vi "Toolkit Binaries Pre-Uninstall Custom Action.vi"(10 "Variant":variant) -> (0 "error out":errorcluster)   [LabVIEW 2020]
uses:
  <vilib>/security/Message Digest/API/Instances/File/SHA-256 File Checksum.vi
  <vilib>/security/Message Digest/API/NI_Message Digest API.lvlib
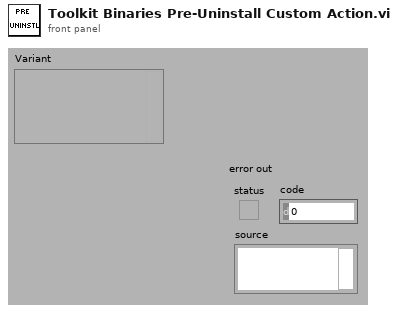
[diagram p1: front panel]
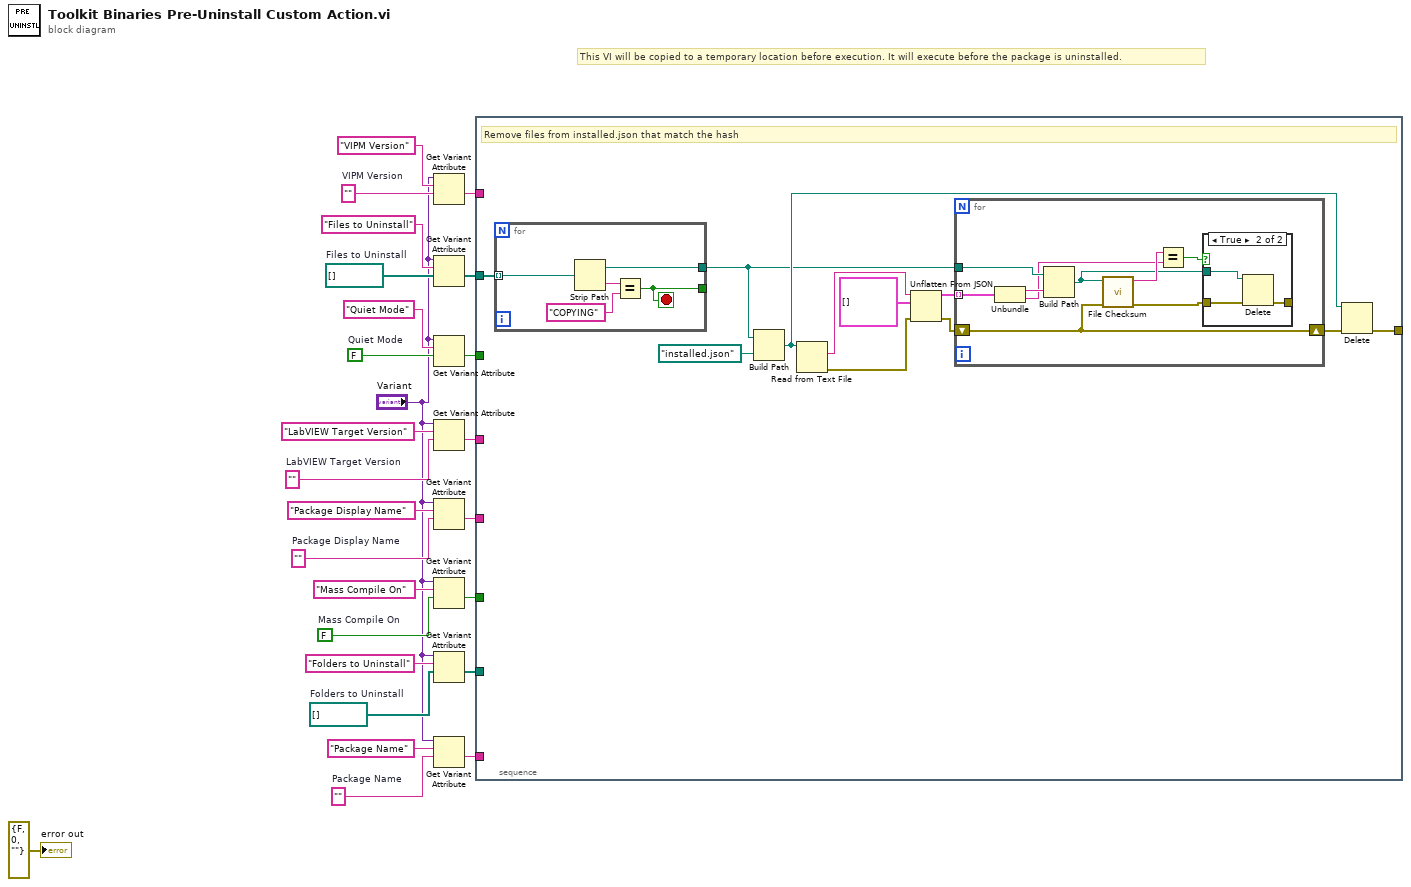
[diagram p0: block diagram]
diagram:
  w3 = path[] []  # Folders to Uninstall
  w7 = path[] []  # Files to Uninstall
  w8 = FALSE  # Mass Compile On
  w9 = ""  # Package Display Name
  w16 = FALSE  # Quiet Mode
  w19 = ""  # VIPM Version
  w21 = ""  # LabVIEW Target Version
  w23 = ""  # Package Name
  # "This VI will be copied to a temporary location before execution. It will execute before the package is uninstalled."
  n1 = Get Variant Attribute(Variant="Variant", name="VIPM Version", default value (empty Variant)=w19) -> (value=w12:string)  [unwired: 1 in, 3 out]
  n2 = Get Variant Attribute(Variant="Variant", name="Files to Uninstall", default value (empty Variant)=w7) -> (value=w5:path[])  [unwired: 1 in, 3 out]
  n3 = Get Variant Attribute(Variant="Variant", name="Quiet Mode", default value (empty Variant)=w16) -> (value=w11:bool)  [unwired: 1 in, 3 out]
  n4 = Get Variant Attribute(Variant="Variant", name="LabVIEW Target Version", default value (empty Variant)=w21) -> (value=w13:string)  [unwired: 1 in, 3 out]
  n5 = Get Variant Attribute(Variant="Variant", name="Package Display Name", default value (empty Variant)=w9) -> (value=w15:string)  [unwired: 1 in, 3 out]
  n6 = Get Variant Attribute(Variant="Variant", name="Mass Compile On", default value (empty Variant)=w8) -> (value=w10:bool)  [unwired: 1 in, 3 out]
  n7 = Get Variant Attribute(Variant="Variant", name="Folders to Uninstall", default value (empty Variant)=w3) -> (value=w2:path[])  [unwired: 1 in, 3 out]
  n8 = Get Variant Attribute(Variant="Variant", name="Package Name", default value (empty Variant)=w23) -> (value=w14:string)  [unwired: 1 in, 3 out]
  n9 = stacked-sequence {
    tunnel: w15 -> [_]
    tunnel: w14 -> [_]
    tunnel: w13 -> [_]
    tunnel: w12 -> [_]
    tunnel: w11 -> [_]
    tunnel: w10 -> [_]
    tunnel: w5 -> [w37]
    tunnel: w2 -> [_]
    tunnel: [w27] -> _
    frame #0 {
      # "Remove files from installed.json that match the hash"
      n10 = for {
        tunnel: w37 -> [w54] mode=indexing
        tunnel: [w51] -> w28
        tunnel: [w50] -> _
        stop <- w50 stop-if-true
        n11 = Strip Path(path=w54) -> (stripped path=w51:path, name=w53:string)
        n12 = Equal?(x=w53, y="COPYING") -> (x = y?=w50:bool)
      }
      n13 = Build Path(base path=w28, name or relative path=path "installed.json") -> (appended path=w29:path)
      n14 = Read from Text File(file (use dialog)=w29) -> (text=w34:string, error out=w35:errorcluster)  [unwired: 3 in, 2 out]
      n15 = Unflatten From JSON(JSON string=w34, type and defaults=cluster{"Path":string, "SHA-256":string}[] [], error in (no error)=w35) -> (value=w32:cluster{"Path":string, "SHA-256":string}[], error out=w31:errorcluster)  [unwired: 4 in]
      n16 = for {
        tunnel: w28 -> [w46]
        tunnel: w32 -> [w45] mode=indexing
        shift-right: [w41] -> w30
        shift-left: w31 -> [w41]
        n17 = Unbundle(w45) -> ("Path"=w44:string, "SHA-256"=w42:string)
        n18 = Build Path(base path=w46, name or relative path=w44) -> (appended path=w38:path)
        n19 = call-poly <vilib>:"File Checksum.vi"("error in"=w41, "path"=w38) -> ("error out"=w40:errorcluster, "digest"=w43:string)  [unwired: 8 in]
        n20 = Equal?(x=w43, y=w42) -> (x = y?=w39:bool)
        n21 = case shown="True" w39 {
          tunnel: w40 -> [_ w49]
          tunnel: [_ w48] -> _
          tunnel: w38 -> [_ w47]
          frame False {
          }
          frame True {
            n22 = Delete(path (use dialog)=w47, error in=w49) -> (error out=w48:errorcluster)  [unwired: 3 in, 2 out]
          }
        }
      }
      n23 = Delete(path (use dialog)=w29, error in=w30) -> (error out=w27:errorcluster)  [unwired: 3 in, 2 out]
    }
  }
  "error out" <- errorcluster {"status"=FALSE, "code"=0, "source"=""} ("error out")
